vi "event.vi"() -> ()   [LabVIEW 2015]
panel:
  in  "OK Button":bool
  out "Numeric 3":dbl
  in  "Numeric 2":dbl
  in  "Numeric":dbl
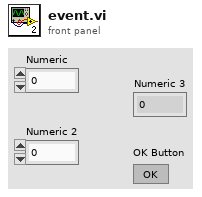
[diagram p1: front panel]
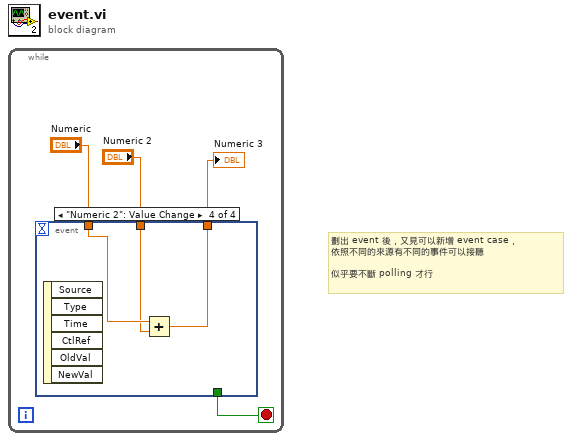
[diagram p0: block diagram]
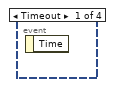
[diagram p2: hidden frame]
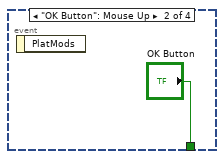
[diagram p3: hidden frame]
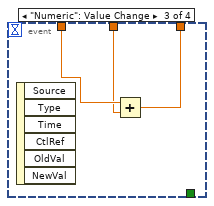
[diagram p4: hidden frame]
diagram:
  # "劃出 event 後，又見可以新增 event case，\n依照不同的來源有不同的事件可以接聽\n\n似乎要不斷 polling 才行"
  n1 = while {
    stop <- w4 stop-if-true
    n2 = event shown="[3] \"Numeric 2\": Value Change" {
      selector: _ -> [_ _ _ _]
      dyn-events: _ -> [_ _ _ _]
      timeout: _ -> [_ _ _ _]
      tunnel: [_ "OK Button" _ _] -> w4
      tunnel: "Numeric" -> [_ _ w8 w11]
      tunnel: "Numeric 2" -> [_ _ w7 w10]
      tunnel: [_ _ w6 w9] -> w1
      event Timeout {
        n3 = event-data() -> ()  [unwired: 1 in, 1 out]
      }
      event "OK Button": Mouse Up {
        n4 = event-data() -> ()  [unwired: 1 in, 1 out]
      }
      event "Numeric": Value Change {
        n5 = event-data() -> ()  [unwired: 1 in, 6 out]
        n6 = Add(x=w8, y=w7) -> (x+y=w6:dbl)
      }
      event "Numeric 2": Value Change {
        n7 = event-data() -> ()  [unwired: 1 in, 6 out]
        n8 = Add(x=w11, y=w10) -> (x+y=w9:dbl)
      }
    }
    "Numeric 3" <- w1
  }
